vi "viewElements.vi"(7 "error in (no error)":errorcluster, 10 "MissionQueue in":refnum<class "MissionQueue.lvclass">) -> (0 "error out":errorcluster, 1 "elements":refnum<class "Mission.lvclass">[](array[class]), 2 "Is empty?":bool, 3 "MissionQueue out":refnum<class "MissionQueue.lvclass">)   [LabVIEW 2011, in "MissionQueue.lvclass"]
uses:
  MissionQueue.lvclass
  Mission/Mission.lvclass
  MissionQueue.lvclass/MissionQueue.ctl
panel:
  out "Queue length":i32
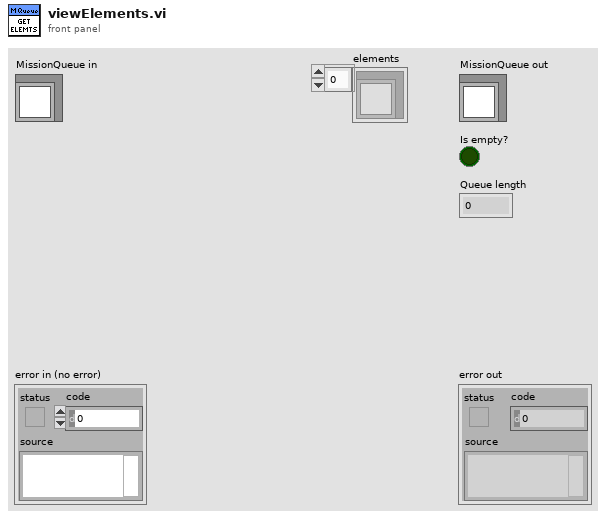
[diagram p1: front panel]
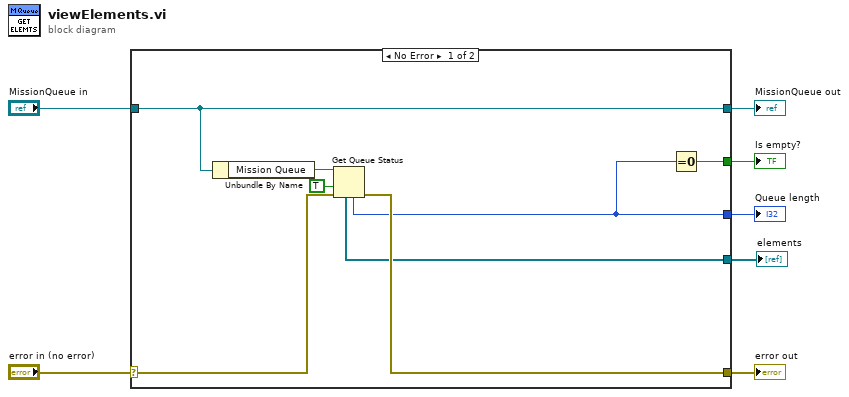
[diagram p0: block diagram]
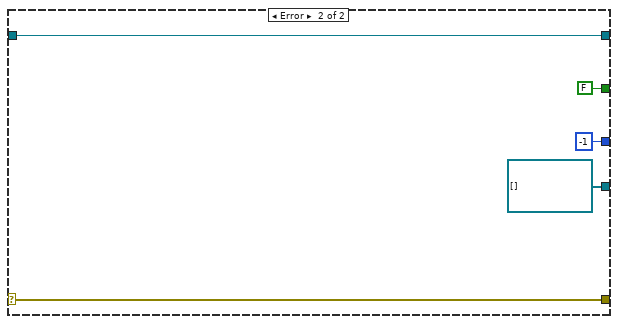
[diagram p2: hidden frame]
diagram:
  n1 = case shown="No Error" "error in (no error)" {
    selector: "error in (no error)" -> [w13 w20]
    tunnel: [w12 w20] -> w6
    tunnel: [w15 w19] -> w4
    tunnel: "MissionQueue in" -> [w15 w19]
    tunnel: [w11 FALSE] -> w3
    tunnel: [w10 -1 ("# elements in queue")] -> w2
    tunnel: [w8 refnum<class "Mission.lvclass">[] [] ("elements")] -> w1
    frame No Error {
      n2 = Unbundle By Name(w15) -> ("Mission Queue"=w14:refnum<queue>)
      n3 = Get Queue Status(queue=w14, return elements? (F)=TRUE, error in (no error)=w13) -> (error out=w12:errorcluster, # elements in queue=w10:i32, elements=w8:refnum<class "Mission.lvclass">[])  [unwired: 5 out]
      n4 = Equal To 0?(x=w10) -> (x = 0?=w11:bool)
    }
    frame Error {
    }
  }
  "error out" <- w6
  "MissionQueue out" <- w4
  "Is empty?" <- w3
  "Queue length" <- w2
  "elements" <- w1
